vi "Set_voltage_Bias.vi"(6 "V step":dbl, 8 "Sweep Spacing_0":string(combo), 9 "Vvar_0_Stop":dbl, 10 "step\nnumber":dbl, 11 "Vvar_0_start":dbl) -> (2 "Vvar":dbl, 3 "nbr steps":dbl)   [LabVIEW 2021]
panel:
  out "String":string
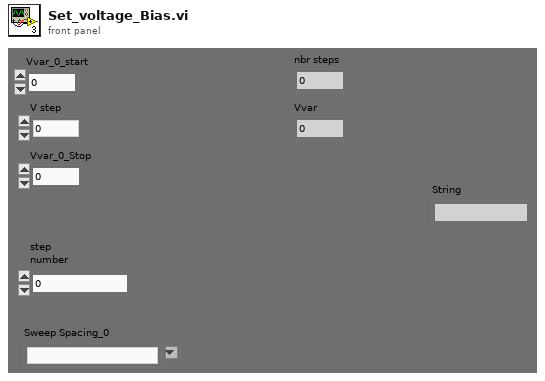
[diagram p1: front panel]
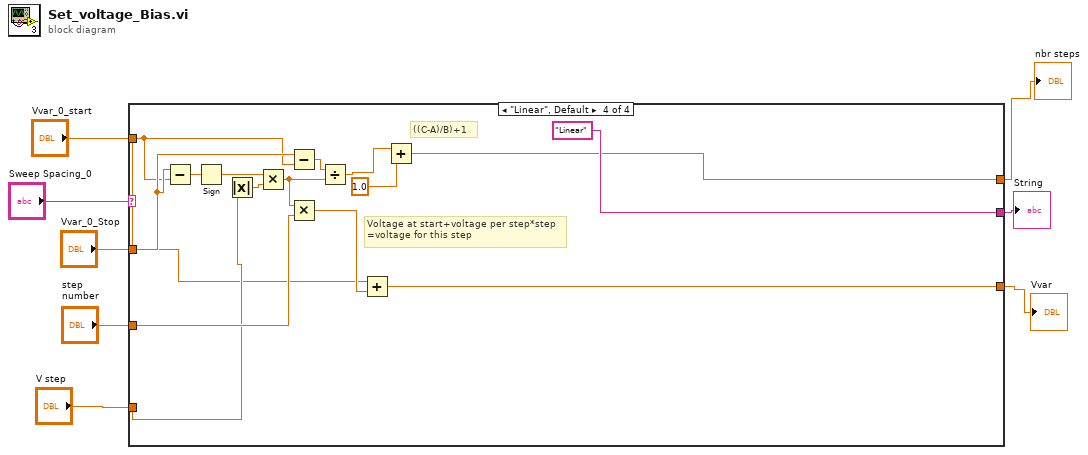
[diagram p0: block diagram]
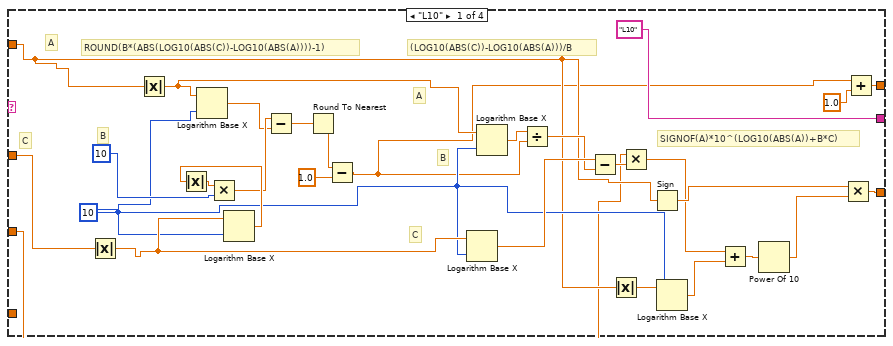
[diagram p2: hidden frame]
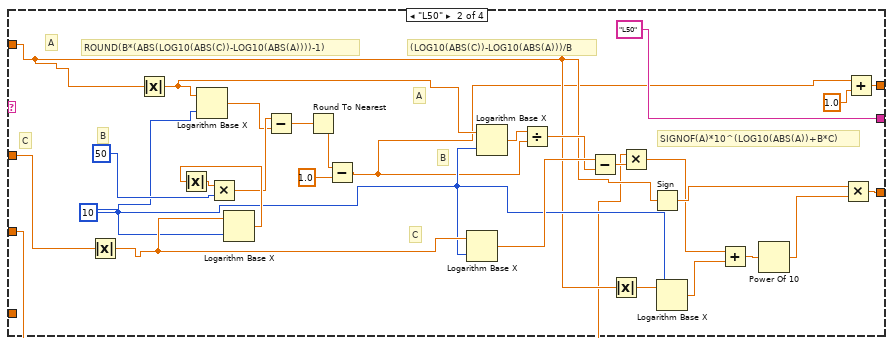
[diagram p3: hidden frame]
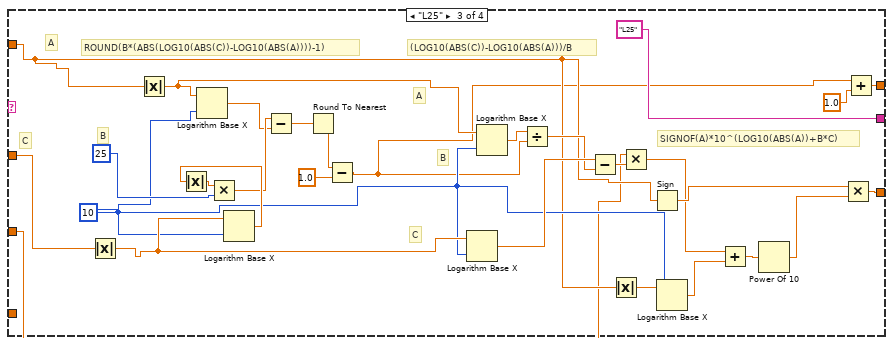
[diagram p4: hidden frame]
diagram:
  n1 = case shown="\"Linear\", Default" "Sweep Spacing_0" {
    tunnel: ["L10" "L50" "L25" "Linear"] -> w7
    tunnel: "step\nnumber" -> [w9 w38 w67 w102]
    tunnel: "Vvar_0_start" -> [w20 w49 w78 w96]
    tunnel: "Vvar_0_Stop" -> [w29 w58 w87 w97]
    tunnel: "V step" -> [_ _ _ w100]
    tunnel: [w10 w39 w68 w99] -> w2
    tunnel: [w13 w42 w71 w98] -> w1
    frame "L10" {
      w21 = 10
      # "SIGNOF(A)*10^(LOG10(ABS(A))+B*C)"
      # "C"
      # "B"
      # "A"
      # "(LOG10(ABS(C))-LOG10(ABS(A)))/B"
      # "C"
      # "B"
      # "A"
      # "ROUND(B*(ABS(LOG10(ABS(C))-LOG10(ABS(A))))-1)"
      n2 = Absolute Value(x=w29) -> (abs(x)=w28:dbl)
      n3 = Absolute Value(x=w20) -> (abs(x)=w27:dbl)
      n4 = Logarithm Base X(1:w21, 2:w27) -> (0:w33:dbl)
      n5 = Logarithm Base X(1:w21, 2:w28) -> (0:w35:dbl)
      n6 = Absolute Value(x=w35) -> (abs(x)=w36:dbl)
      n7 = Multiply(x=w36, y=10) -> (x*y=w34:dbl)
      n8 = Subtract(x=w34, y=w33) -> (x-y=w32:dbl)
      n9 = Round To Nearest(number=w32) -> (nearest integer value=w30:dbl)
      n10 = Subtract(x=w30, y=1.0) -> (x-y=w11:dbl)
      n11 = Logarithm Base X(1:w21, 2:w28) -> (0:w25:dbl)
      n12 = Logarithm Base X(1:w21, 2:w27) -> (0:w26:dbl)
      n13 = Divide(x=w26, y=w11) -> (x/y=w24:dbl)
      n14 = Subtract(x=w25, y=w24) -> (x-y=w16:dbl)
      n15 = Absolute Value(x=w20) -> (abs(x)=w19:dbl)
      n16 = Multiply(x=w9, y=w16) -> (x*y=w17:dbl)
      n17 = Sign(1:w20) -> (0:w22:dbl)
      n18 = Logarithm Base X(1:w21, 2:w19) -> (0:w18:dbl)
      n19 = Add(x=w17, y=w18) -> (x+y=w15:dbl)
      n20 = Power Of 10(x=w15) -> (10^x=w14:dbl)
      n21 = Multiply(x=w22, y=w14) -> (x*y=w13:dbl)
      n22 = Add(x=w11, y=1.0) -> (x+y=w10:dbl)
    }
    frame "L50" {
      w50 = 10
      # "SIGNOF(A)*10^(LOG10(ABS(A))+B*C)"
      # "C"
      # "B"
      # "A"
      # "(LOG10(ABS(C))-LOG10(ABS(A)))/B"
      # "C"
      # "B"
      # "A"
      # "ROUND(B*(ABS(LOG10(ABS(C))-LOG10(ABS(A))))-1)"
      n23 = Absolute Value(x=w58) -> (abs(x)=w57:dbl)
      n24 = Absolute Value(x=w49) -> (abs(x)=w56:dbl)
      n25 = Logarithm Base X(1:w50, 2:w56) -> (0:w62:dbl)
      n26 = Logarithm Base X(1:w50, 2:w57) -> (0:w64:dbl)
      n27 = Absolute Value(x=w64) -> (abs(x)=w65:dbl)
      n28 = Multiply(x=w65, y=50) -> (x*y=w63:dbl)
      n29 = Subtract(x=w63, y=w62) -> (x-y=w61:dbl)
      n30 = Round To Nearest(number=w61) -> (nearest integer value=w59:dbl)
      n31 = Subtract(x=w59, y=1.0) -> (x-y=w40:dbl)
      n32 = Logarithm Base X(1:w50, 2:w57) -> (0:w54:dbl)
      n33 = Logarithm Base X(1:w50, 2:w56) -> (0:w55:dbl)
      n34 = Divide(x=w55, y=w40) -> (x/y=w53:dbl)
      n35 = Subtract(x=w54, y=w53) -> (x-y=w45:dbl)
      n36 = Absolute Value(x=w49) -> (abs(x)=w48:dbl)
      n37 = Multiply(x=w38, y=w45) -> (x*y=w46:dbl)
      n38 = Sign(1:w49) -> (0:w51:dbl)
      n39 = Logarithm Base X(1:w50, 2:w48) -> (0:w47:dbl)
      n40 = Add(x=w46, y=w47) -> (x+y=w44:dbl)
      n41 = Power Of 10(x=w44) -> (10^x=w43:dbl)
      n42 = Multiply(x=w51, y=w43) -> (x*y=w42:dbl)
      n43 = Add(x=w40, y=1.0) -> (x+y=w39:dbl)
    }
    frame "L25" {
      w79 = 10
      # "SIGNOF(A)*10^(LOG10(ABS(A))+B*C)"
      # "C"
      # "B"
      # "A"
      # "(LOG10(ABS(C))-LOG10(ABS(A)))/B"
      # "C"
      # "B"
      # "A"
      # "ROUND(B*(ABS(LOG10(ABS(C))-LOG10(ABS(A))))-1)"
      n44 = Absolute Value(x=w87) -> (abs(x)=w86:dbl)
      n45 = Absolute Value(x=w78) -> (abs(x)=w85:dbl)
      n46 = Logarithm Base X(1:w79, 2:w85) -> (0:w91:dbl)
      n47 = Logarithm Base X(1:w79, 2:w86) -> (0:w93:dbl)
      n48 = Absolute Value(x=w93) -> (abs(x)=w94:dbl)
      n49 = Multiply(x=w94, y=25) -> (x*y=w92:dbl)
      n50 = Subtract(x=w92, y=w91) -> (x-y=w90:dbl)
      n51 = Round To Nearest(number=w90) -> (nearest integer value=w88:dbl)
      n52 = Subtract(x=w88, y=1.0) -> (x-y=w69:dbl)
      n53 = Logarithm Base X(1:w79, 2:w86) -> (0:w83:dbl)
      n54 = Logarithm Base X(1:w79, 2:w85) -> (0:w84:dbl)
      n55 = Divide(x=w84, y=w69) -> (x/y=w82:dbl)
      n56 = Subtract(x=w83, y=w82) -> (x-y=w74:dbl)
      n57 = Absolute Value(x=w78) -> (abs(x)=w77:dbl)
      n58 = Multiply(x=w67, y=w74) -> (x*y=w75:dbl)
      n59 = Sign(1:w78) -> (0:w80:dbl)
      n60 = Logarithm Base X(1:w79, 2:w77) -> (0:w76:dbl)
      n61 = Add(x=w75, y=w76) -> (x+y=w73:dbl)
      n62 = Power Of 10(x=w73) -> (10^x=w72:dbl)
      n63 = Multiply(x=w80, y=w72) -> (x*y=w71:dbl)
      n64 = Add(x=w69, y=1.0) -> (x+y=w68:dbl)
    }
    frame "Linear", Default {
      # "Voltage at start+voltage per step*step\n=voltage for this step"
      # "((C-A)/B)+1"
      n65 = Subtract(x=w97, y=w96) -> (x-y=w103:dbl)
      n66 = Sign(1:w103) -> (0:w104:dbl)
      n67 = Absolute Value(x=w100) -> (abs(x)=w105:dbl)
      n68 = Multiply(x=w104, y=w105) -> (x*y=w109:dbl)
      n69 = Subtract(x=w97, y=w96) -> (x-y=w106:dbl)
      n70 = Multiply(x=w109, y=w102) -> (x*y=w108:dbl)
      n71 = Divide(x=w106, y=w109) -> (x/y=w107:dbl)
      n72 = Add(x=w96, y=w108) -> (x+y=w98:dbl)
      n73 = Add(x=w107, y=1.0) -> (x+y=w99:dbl)
    }
  }
  "String" <- w7
  "nbr steps" <- w2
  "Vvar" <- w1
